vi "TestBed.vi"() -> ()   [LabVIEW 2015]
uses:
  S2C_XML_Globals.vi
  <vilib>/xml/Close Reference(Node).vi
  <vilib>/xml/NI_XML.lvlib
  <resource>/objmgr/DOMUserDefRef.rc
panel:
  in  "TestData":T1={"TestName"="JSWUpdate_Tests", "TestDateTime"="2024-09-19 09:02:11.570", "TestStatus"="", "Comment"=""}
  in  "MeasMeta":cluster{"MetaName":string, "MetaValue":string}[](array[cluster])=[{"MetaName"="GTIN_External", "MetaValue"="10884521829527"}, {"MetaName"="Shift", "MetaValue"="1"}]
  in  "MeasData":T2(array[cluster])=[{"MeasName"="MyStringTest", "MeasDateTime"="2024-09-19 09:02:11.570", "Comment"="", "MeasType"="String", "MeasValue"="Test", "TargetValue"="Test", "HL Comp"="", "HighLimit"="", "LL Comp"="", "LowLimit"="", "Units"="None", "MeasStatus"="Passed"}]
  in  "EventData":T3={"EventName"="Hardware_JSWUpdate_Event", "ProcessName"="Manufacturing", "ProductLine"="Hardware", "EventStatus"="", "EventStart"="2024-09-19 09:01:35.665", "EventStop"="", "Station"="HW_JSWUpdate1", "OperatorName"="1234", "Location"=""}
  in  "EventMeta":cluster{"MetaName":string, "MetaValue":string}[](array[cluster])=[{"MetaName"="GTIN_External", "MetaValue"="10884521829527"}, {"MetaName"="Shift", "MetaValue"="1"}]
  in  "AssetData":T4={"SN"="T1A00030DX", "Manufacturer"="Medtronic", "Model"="VLFT10FXGEN"}
  out "XML Output":string
  out "Error Out":errorcluster
  in  "Error In":errorcluster
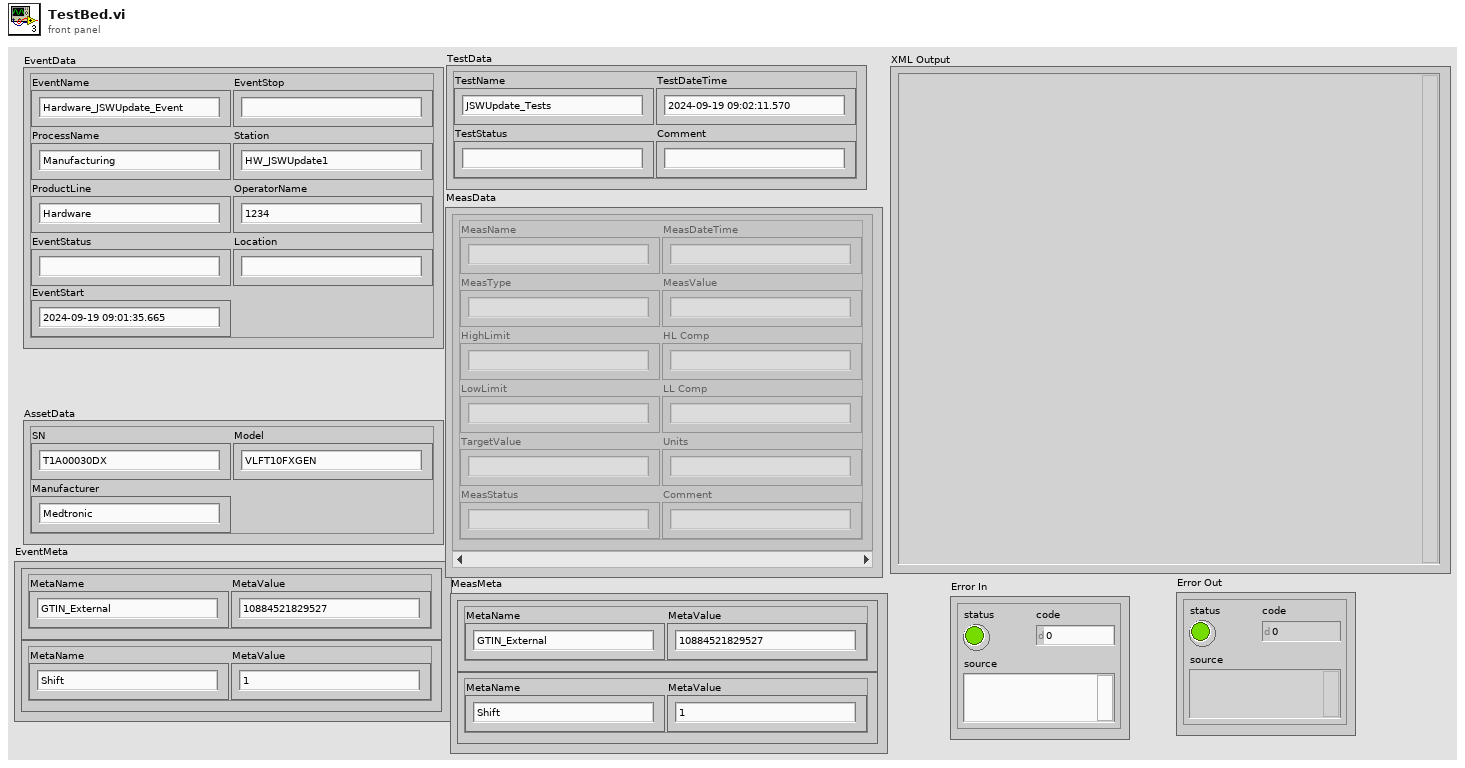
[diagram p1: front panel]
types:
  T1 = cluster{"TestName":string, "TestDateTime":string, "TestStatus":string, "Comment":string}
  T2 = cluster{"MeasName":string, "MeasDateTime":string, "Comment":string, "MeasType":string, "MeasValue":string, "TargetValue":string, "HL Comp":string, "HighLimit":string, "LL Comp":string, "LowLimit":string, "Units":string, "MeasStatus":string}[]
  T3 = cluster{"EventName":string, "ProcessName":string, "ProductLine":string, "EventStatus":string, "EventStart":string, "EventStop":string, "Station":string, "OperatorName":string, "Location":string}
  T4 = cluster{"SN":string, "Manufacturer":string, "Model":string}
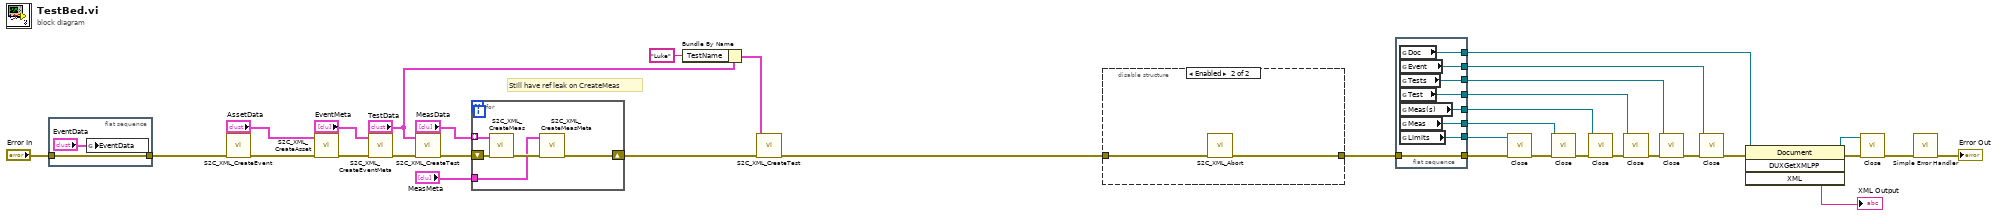
[diagram p0: block diagram]
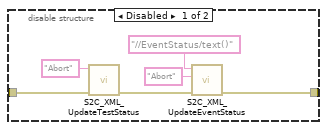
[diagram p2: hidden frame]
diagram:
  # "Still have ref leak on CreateMeas"
  n1 = flat-sequence {
    tunnel: "Error In" -> [w36]
    tunnel: [w36] -> w8
    frame #0 {
      n2 = global write "S2C_XML_Globals.vi" "EventData"("EventData") -> ()
    }
  }
  n3 = call "S2C_XML_CreateEvent.vi"("Error In"=w8) -> ("Error Out"=w14:errorcluster)  [unwired: 10 in]
  n4 = call "S2C_XML_CreateAsset.vi"("Error In"=w14, "AssetData"="AssetData") -> ("Error Out"=w12:errorcluster)  [unwired: 9 in]
  n5 = call "S2C_XML_CreateEventMeta.vi"("Error In"=w12, "MetaArray"="EventMeta") -> ("Error Out"=w10:errorcluster)  [unwired: 9 in]
  n6 = call "S2C_XML_CreateTest.vi"("Error In"=w10, "TestData"="TestData") -> ("Error Out"=w9:errorcluster)  [unwired: 9 in]
  n7 = for {
    shift-right: [w38] -> w4
    shift-left: w9 -> [w42]
    tunnel: "MeasData" -> [w41] mode=indexing
    tunnel: "MeasMeta" -> [w39]
    n8 = call "S2C_XML_CreateMeas.vi"("Error In"=w42, "MeasData"=w41) -> ("Error Out"=w40:errorcluster)  [unwired: 9 in]
    n9 = call "S2C_XML_CreateMeasMeta.vi"("Error In"=w40, "MetaArray"=w39) -> ("Error Out"=w38:errorcluster)  [unwired: 9 in]
  }
  n10 = Bundle By Name(cluster="TestData", "TestName"="Luke") -> (w2:T1)
  n11 = call "S2C_XML_CreateTest.vi"("Error In"=w4, "TestData"=w2) -> ("Error Out"=w1:errorcluster)  [unwired: 9 in]
  n12 = disable-structure shown="Enabled" {
    disable-tunnel: w1 -> [w48 w49]
    disable-tunnel: [w45 w50] -> w18
    frame Disabled {
      n13 = call "S2C_XML_UpdateTestStatus.vi"("Error In"=w48, "Result"="Abort") -> ("Error Out"=w46:errorcluster)  [unwired: 9 in]
      n14 = call "S2C_XML_UpdateEventStatus.vi"("Error In"=w46, 10:"Abort" ("Value"), "Value"="//EventStatus/text()" ("Xpath")) -> ("Error Out"=w45:errorcluster)  [unwired: 8 in]
    }
    frame Enabled {
      n15 = call "S2C_XML_Abort.vi"("Error In"=w49) -> ("Error Out"=w50:errorcluster)  [unwired: 10 in]
    }
  }
  n16 = flat-sequence {
    tunnel: w18 -> [w56]
    tunnel: [w58] -> w29
    tunnel: [w57] -> w28
    tunnel: [w56] -> w17
    tunnel: [w55] -> w27
    tunnel: [w54] -> w25
    tunnel: [w53] -> w21
    tunnel: [w52] -> w20
    tunnel: [w51] -> w15
    frame #0 {
      n17 = global read "S2C_XML_Globals.vi" "Doc"() -> (w57:refnum<k20>)
      n18 = global read "S2C_XML_Globals.vi" "Event"() -> (w58:refnum<k20>)
      n19 = global read "S2C_XML_Globals.vi" "Tests"() -> (w55:refnum<k20>)
      n20 = global read "S2C_XML_Globals.vi" "Test"() -> (w54:refnum<k20>)
      n21 = global read "S2C_XML_Globals.vi" "Meas(s)"() -> (w53:refnum<k20>)
      n22 = global read "S2C_XML_Globals.vi" "Meas"() -> (w52:refnum<k20>)
      n23 = global read "S2C_XML_Globals.vi" "Limits"() -> (w51:refnum<k20>)
    }
  }
  n24 = call-poly <vilib>:"Close.vi"("error in (no error)"=w17, "node"=w15) -> ("error out"=w16:errorcluster)  [unwired: 7 in]
  n25 = call-poly <vilib>:"Close.vi"("error in (no error)"=w16, "node"=w20) -> ("error out"=w23:errorcluster)  [unwired: 7 in]
  n26 = call-poly <vilib>:"Close.vi"("error in (no error)"=w23, "node"=w21) -> ("error out"=w22:errorcluster)  [unwired: 7 in]
  n27 = call-poly <vilib>:"Close.vi"("error in (no error)"=w22, "node"=w25) -> ("error out"=w24:errorcluster)  [unwired: 7 in]
  n28 = call-poly <vilib>:"Close.vi"("error in (no error)"=w24, "node"=w27) -> ("error out"=w26:errorcluster)  [unwired: 7 in]
  n29 = call-poly <vilib>:"Close.vi"("error in (no error)"=w26, "node"=w29) -> ("error out"=w35:errorcluster)  [unwired: 7 in]
  n30 = invoke class="Document" method="DUXGetXMLPP"(reference=w28, error in=w35) -> (reference out=w32:refnum<k20>, error out=w33:errorcluster, "XML"=→"XML Output":string)  [unwired: 2 in, 1 out]
  n31 = call-poly <vilib>:"Close.vi"("error in (no error)"=w33, "node"=w32) -> ("error out"=w31:errorcluster)  [unwired: 7 in]
  n32 = call <vilib>:"Simple Error Handler.vi"("error in (no error)"=w31) -> ("error out"=→"Error Out":errorcluster)  [unwired: 4 in, 4 out]
